vi "Initialize.vi"(8 "error in":errorcluster, 11 "Modbus master in":refnum<class "Modbus Master.lvclass">) -> (0 "error out":errorcluster, 3 "Modbus master out":refnum<class "Modbus Master.lvclass">)   [LabVIEW 2012, in "Modbus Master.lvclass"]
doc: "Initializes a Modbus master instance. If using the <B>Create Modbus Instance</B> VI, this is not necessary. This function will initiate any required bus communication."
uses:
  Modbus Master.lvclass
  Modbus Master.lvclass/Modbus Master.ctl
  Network Protocol/Network Master/Network Master.lvclass
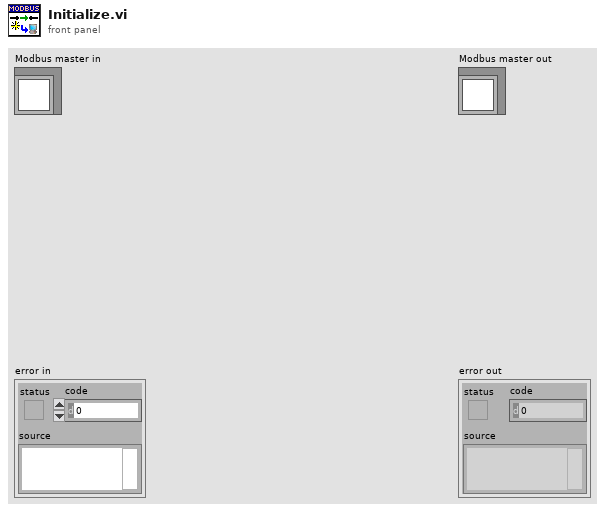
[diagram p1: front panel]
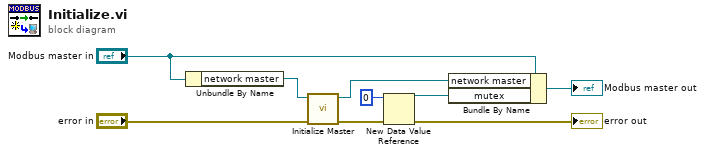
[diagram p0: block diagram]
diagram:
  n1 = Unbundle By Name("Modbus master in") -> ("network master"=w5:refnum<class "Network Master.lvclass">)
  n2 = call-dynamic "Initialize Master.vi"("error in"="error in", "Network Master in"=w5) -> ("error out"=w4:errorcluster, "Network Master out"=w8:refnum<class "Network Master.lvclass">)  [unwired: 8 in]
  n3 = New Data Value Reference(data value=u8 0, error in=w4) -> (data value reference=w2:refnum<data-value>, error out=→"error out":errorcluster)
  n4 = Bundle By Name(cluster="Modbus master in", "network master"=w8, "mutex"=w2) -> (→"Modbus master out":refnum<class "Modbus Master.lvclass">)
